vi "InstrumentSelection.vi"(8 "error in (no error)":errorcluster, 9 "Verify GPIB address":bool, 10 "Instrument type":T1(ring), 11 "Instrument name IN":string(combo)) -> (0 "error out":errorcluster, 1 "Instrument name OUT":string, 2 "LCR":refnum<class "LCRControl.lvclass">, 3 "Supply":refnum<class "SupplyControl.lvclass">, 4 "Switching":refnum<class "Switching.lvclass">, 5 "Multimeter":refnum<class "MultimeterControl.lvclass">)   [LabVIEW 2018, in "InstrControl.lvclass"]
uses:
  InstrControl.lvclass
  SupplyControl/SupplyControl.lvclass
  C:/Users/itk/Documents/itk-strip-sensor-qc/InstrControl/InstrControl.lvclass
  LCRControl/LCRControl.lvclass
  MultimeterControl/MultimeterControl.lvclass
  Switching/Switching.lvclass
  SupplyControl/Keithley 2410/KE2410.lvclass
  C:/Users/itk/Documents/itk-strip-sensor-qc/InstrControl/SupplyControl/SupplyControl.lvclass
  SupplyControl/Keithley 6517/KE6517.lvclass
  SupplyControl/Keithley 487/KE487.lvclass
  SupplyControl/Keithley 2657/KE2657A.lvclass
  SupplyControl/Keithley 236 & 237/KE236.lvclass
  LCRControl/WK6440B/WK6440B.lvclass
  C:/Users/itk/Documents/itk-strip-sensor-qc/InstrControl/LCRControl/LCRControl.lvclass
  LCRControl/WK6425/WK6425.lvclass
  MultimeterControl/Keithley 2000/KE2000.lvclass
  C:/Users/itk/Documents/itk-strip-sensor-qc/InstrControl/MultimeterControl/MultimeterControl.lvclass
  Switching/Pickering/Pickering.lvclass
  C:/Users/itk/Documents/itk-strip-sensor-qc/InstrControl/Switching/Switching.lvclass
  InstrumentSetup.vi
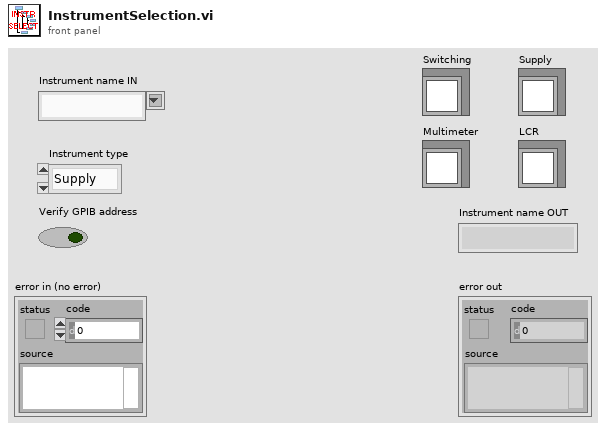
[diagram p1: front panel]
types:
  T1 = enum16{"Supply", "LCR", "Multimeter", "Switching"}
  T2 = cluster{"KE 2410":cluster{"Instrument name":string, "GPIB address":string, "Instrument type":u16}, "KE 6517":cluster{"Instrument name":string, "GPIB address":string, "Instrument type":u16}, "KE 487":cluster{"Instrument name":string, "GPIB address":string, "Instrument type":u16}, "KE 487_2":cluster{"Instrument name":string, "GPIB address":string, "Instrument type":u16}, "KE 236":cluster{"Instrument name":string, "GPIB address":string, "Instrument type":u16}, "WK 6440B":cluster{"Instrument name":string, "GPIB address":string, "Instrument type":u16}, "WK 6425":cluster{"Instrument name":string, "GPIB address":string, "Instrument type":u16}, "Pickering Matrix":cluster{"Instrument name":string, "GPIB address":string, "Instrument type":u16}, "KE 2000":cluster{"Instrument name":string, "GPIB address":string, "Instrument type":u16}, "KE 2657A":cluster{"Instrument name":string, "GPIB address":string, "Instrument type":u16}, "Prague Pickering Matrix":cluster{"Instrument name":string, "GPIB address":string, "Instrument type":u16}}
  T3 = cluster{"Current Limit":sgl, "KE2410":refnum<class "KE2410.lvclass">}
  T4 = cluster{"Current Limit":u16, "KE6517":refnum<class "KE6517.lvclass">}
  T5 = cluster{"Compliance":u16, "Range:":u16, "KE487":refnum<class "KE487.lvclass">}
  T6 = cluster{"Current Limit":sgl, "Compliance":u16, "Range:":u16, "KE2657A":refnum<class "KE2657A.lvclass">}
  T7 = cluster{"current \ncompliance level":dbl, "compliance/\nmeasurement range (auto:0)":u16, "KE236":refnum<class "KE236.lvclass">}
  T8 = cluster{"RC Configuration":u16, "AC amplitude [V]":dbl, "AC frequency [Hz]":i32, "WK6440B":refnum<class "WK6440B.lvclass">}
  T9 = cluster{"RC Configuration":u16, "AC amplitude [V]":dbl, "AC frequency [Hz]":i32, "WK6425":refnum<class "WK6425.lvclass">}
  T10 = cluster{"Range":u16, "Range Value":dbl, "Function":u16, "KE2000":refnum<class "KE2000.lvclass">}
  T11 = cluster{"Matrix address":string, "Mux1 address":string, "Mux2 address":string, "Matrix used?":bool, "Pickering":refnum<class "Pickering.lvclass">, "Matrix X Channels":cluster{"Bias Supply / SMU LO":i32, "Bias Supply / SMU HI":i32, "CV Box LO":i32, "CV Box HI":i32, "CV Box LO IN":i32, "CV Box HI IN":i32, "Volt meter LO":i32, "Volt meter HI":i32, "Mux1 C1":i32, "Mux1 C2":i32, "Mux2 C1":i32, "Mux2 C2":i32}}
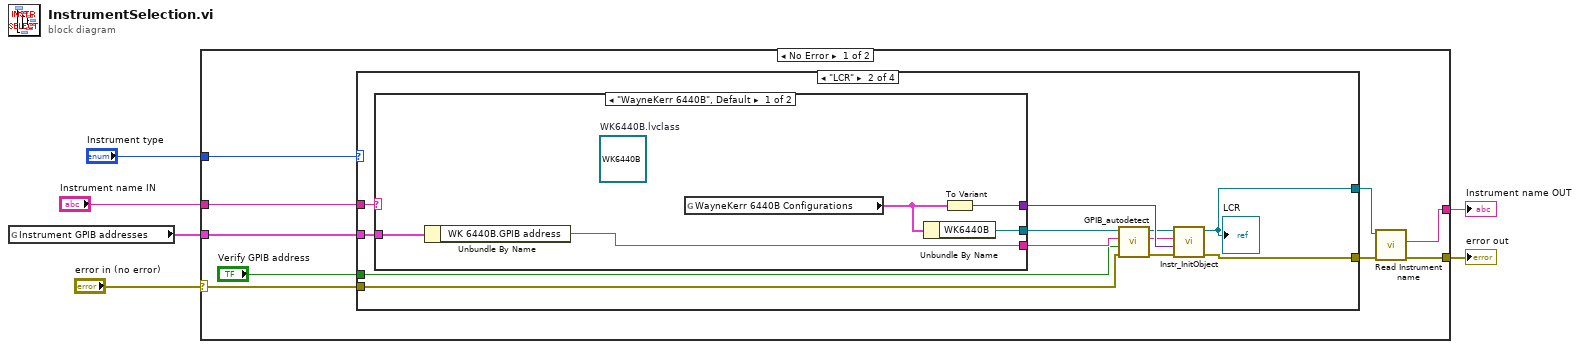
[diagram p0: block diagram]
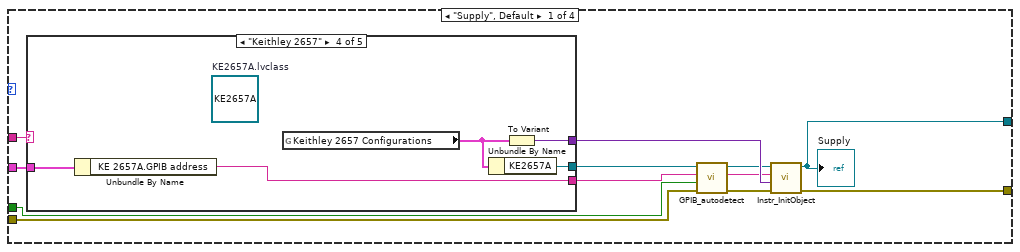
[diagram p2: hidden frame]
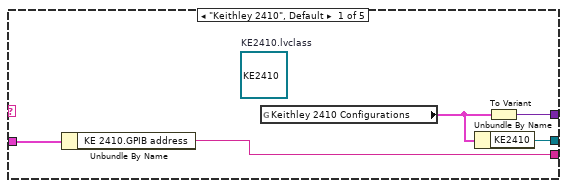
[diagram p3: hidden frame]
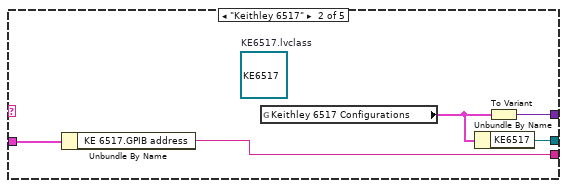
[diagram p4: hidden frame]
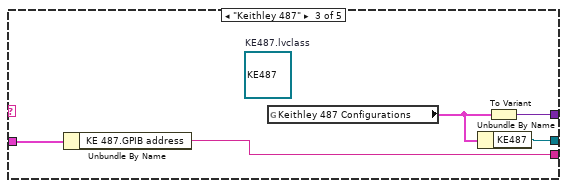
[diagram p5: hidden frame]
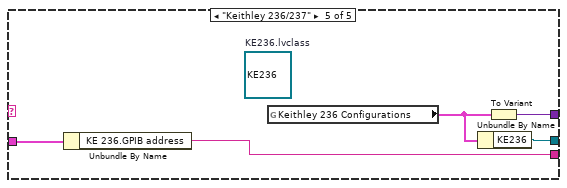
[diagram p6: hidden frame]
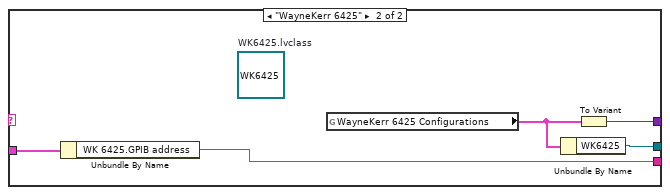
[diagram p7: hidden frame]
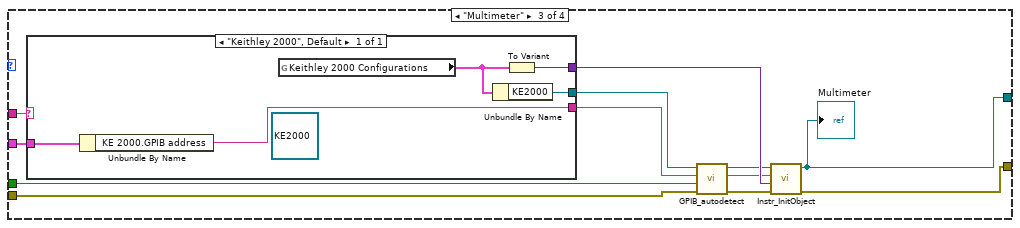
[diagram p8: hidden frame]
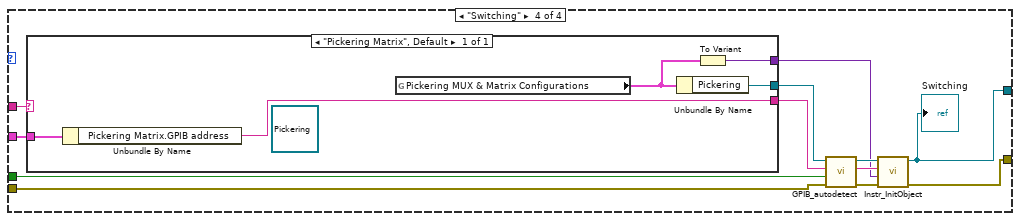
[diagram p9: hidden frame]
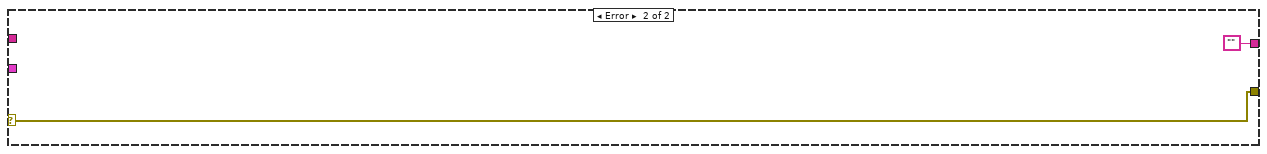
[diagram p10: hidden frame]
diagram:
  n1 = global read "InstrumentSetup.vi" "Instrument GPIB addresses"() -> (w1:T2)
  n2 = case shown="No Error" "error in (no error)" {
    selector: "error in (no error)" -> [w13 w110]
    tunnel: [w14 w110] -> w5
    tunnel: [w15 ""] -> w4
    tunnel: "Instrument type" -> [w10 _]
    tunnel: "Instrument name IN" -> [w9 _]
    tunnel: w1 -> [w8 _]
    frame No Error {
      n3 = case shown="\"LCR\"" w10 {
        tunnel: w9 -> [w27 w64 w86 w94]
        tunnel: [w26 w62 w84 w102] -> w12
        tunnel: w13 -> [w18 w59 w76 w96]
        tunnel: [w25 w63 w85 w103] -> w11
        tunnel: w8 -> [w24 w61 w83 w100]
        tunnel: "Verify GPIB address" -> [w17 w53 w81 w95]
        frame "Supply", Default {
          n4 = case shown="\"Keithley 2657\"" w27 {
            tunnel: [w29 w33 w38 w43 w48] -> w20
            tunnel: w24 -> [w32 w37 w42 w47 w52]
            tunnel: [w31 w36 w41 w46 w51] -> w22
            tunnel: [w30 w35 w40 w45 w50] -> w23
            frame "Keithley 2410", Default {
              (unwired) refnum<class "KE2410.lvclass"> refnum  # KE2410.lvclass
              n5 = Unbundle By Name(w32) -> ("KE 2410.GPIB address"=w31:string)
              n6 = global read "InstrumentSetup.vi" "Keithley 2410 Configurations"() -> (w28:T3)
              n7 = Unbundle By Name(w28) -> ("KE2410"=w29:refnum<class "KE2410.lvclass">)
              n8 = To Variant(anything=w28) -> (Variant=w30:variant)
            }
            frame "Keithley 6517" {
              (unwired) refnum<class "KE6517.lvclass"> refnum  # KE6517.lvclass
              n9 = Unbundle By Name(w37) -> ("KE 6517.GPIB address"=w36:string)
              n10 = global read "InstrumentSetup.vi" "Keithley 6517 Configurations"() -> (w34:T4)
              n11 = Unbundle By Name(w34) -> ("KE6517"=w33:refnum<class "KE6517.lvclass">)
              n12 = To Variant(anything=w34) -> (Variant=w35:variant)
            }
            frame "Keithley 487" {
              (unwired) refnum<class "KE487.lvclass"> refnum  # KE487.lvclass
              n13 = Unbundle By Name(w42) -> ("KE 487.GPIB address"=w41:string)
              n14 = global read "InstrumentSetup.vi" "Keithley 487 Configurations"() -> (w39:T5)
              n15 = Unbundle By Name(w39) -> ("KE487"=w38:refnum<class "KE487.lvclass">)
              n16 = To Variant(anything=w39) -> (Variant=w40:variant)
            }
            frame "Keithley 2657" {
              (unwired) refnum<class "KE2657A.lvclass"> refnum  # KE2657A.lvclass
              n17 = Unbundle By Name(w47) -> ("KE 2657A.GPIB address"=w46:string)
              n18 = global read "InstrumentSetup.vi" "Keithley 2657 Configurations"() -> (w44:T6)
              n19 = Unbundle By Name(w44) -> ("KE2657A"=w43:refnum<class "KE2657A.lvclass">)
              n20 = To Variant(anything=w44) -> (Variant=w45:variant)
            }
            frame "Keithley 236/237" {
              (unwired) refnum<class "KE236.lvclass"> refnum  # KE236.lvclass
              n21 = Unbundle By Name(w52) -> ("KE 236.GPIB address"=w51:string)
              n22 = global read "InstrumentSetup.vi" "Keithley 236 Configurations"() -> (w49:T7)
              n23 = Unbundle By Name(w49) -> ("KE236"=w48:refnum<class "KE236.lvclass">)
              n24 = To Variant(anything=w49) -> (Variant=w50:variant)
            }
          }
          n25 = call-dynamic "GPIB_autodetect.vi"("error in (no error)"=w18, "Verify GPIB address"=w17, "Instrument GPIB address in"=w22, "InstrControl in"=w20) -> ("error out"=w16:errorcluster, "Instrument GPIB address"=w21:string, "InstrControl out"=w19:refnum<class "SupplyControl.lvclass">)  [unwired: 5 in]
          n26 = call-dynamic "Instr_InitObject.vi"("error in (no error)"=w16, "Instrument Configuration"=w23, "GPIB address"=w21, "SupplyControl in"=w19) -> ("error out"=w25:errorcluster, "SupplyControl out"=w26:refnum<class "SupplyControl.lvclass">)  [unwired: 6 in]
          "Supply" <- w26
        }
        frame "LCR" {
          n27 = case shown="\"WayneKerr 6440B\", Default" w64 {
            tunnel: [w65 w70] -> w55
            tunnel: w61 -> [w69 w74]
            tunnel: [w68 w73] -> w57
            tunnel: [w67 w72] -> w60
            frame "WayneKerr 6440B", Default {
              (unwired) refnum<class "WK6440B.lvclass"> refnum  # WK6440B.lvclass
              n28 = Unbundle By Name(w69) -> ("WK 6440B.GPIB address"=w68:string)
              n29 = global read "InstrumentSetup.vi" "WayneKerr 6440B Configurations"() -> (w66:T8)
              n30 = Unbundle By Name(w66) -> ("WK6440B"=w65:refnum<class "WK6440B.lvclass">)
              n31 = To Variant(anything=w66) -> (Variant=w67:variant)
            }
            frame "WayneKerr 6425" {
              (unwired) refnum<class "WK6425.lvclass"> refnum  # WK6425.lvclass
              n32 = Unbundle By Name(w74) -> ("WK 6425.GPIB address"=w73:string)
              n33 = global read "InstrumentSetup.vi" "WayneKerr 6425 Configurations"() -> (w71:T9)
              n34 = Unbundle By Name(w71) -> ("WK6425"=w70:refnum<class "WK6425.lvclass">)
              n35 = To Variant(anything=w71) -> (Variant=w72:variant)
            }
          }
          n36 = call-dynamic "GPIB_autodetect.vi"("error in (no error)"=w59, "Verify GPIB address"=w53, "Instrument GPIB address in"=w57, "InstrControl in"=w55) -> ("error out"=w58:errorcluster, "Instrument GPIB address"=w56:string, "InstrControl out"=w54:refnum<class "LCRControl.lvclass">)  [unwired: 5 in]
          n37 = call-dynamic "Instr_InitObject.vi"("error in (no error)"=w58, "Instrument Configuration"=w60, "GPIB Address"=w56, "LCRControl in"=w54) -> ("error out"=w63:errorcluster, "LCRControl out"=w62:refnum<class "LCRControl.lvclass">)  [unwired: 6 in]
          "LCR" <- w62
        }
        frame "Multimeter" {
          n38 = case shown="\"Keithley 2000\", Default" w86 {
            tunnel: [w87] -> w77
            tunnel: w83 -> [w91]
            tunnel: [w90] -> w80
            tunnel: [w89] -> w82
            frame "Keithley 2000", Default {
              (unwired) refnum<class "KE2000.lvclass"> refnum ("KE2000.lvclass")
              n39 = Unbundle By Name(w91) -> ("KE 2000.GPIB address"=w90:string)
              n40 = global read "InstrumentSetup.vi" "Keithley 2000 Configurations"() -> (w88:T10)
              n41 = Unbundle By Name(w88) -> ("KE2000"=w87:refnum<class "KE2000.lvclass">)
              n42 = To Variant(anything=w88) -> (Variant=w89:variant)
            }
          }
          n43 = call-dynamic "GPIB_autodetect.vi"("error in (no error)"=w76, "Verify GPIB address"=w81, "Instrument GPIB address in"=w80, "InstrControl in"=w77) -> ("error out"=w75:errorcluster, "Instrument GPIB address"=w79:string, "InstrControl out"=w78:refnum<class "KE2000.lvclass">)  [unwired: 5 in]
          n44 = call-dynamic "Instr_InitObject.vi"("error in (no error)"=w75, "Instrument Configuration"=w82, "GPIB Address"=w79, "KE2000 in"=w78) -> ("error out"=w85:errorcluster, "KE2000 out"=w84:refnum<class "KE2000.lvclass">)  [unwired: 6 in]
          "Multimeter" <- w84
        }
        frame "Switching" {
          n45 = case shown="\"Pickering Matrix\", Default" w94 {
            tunnel: w100 -> [w108]
            tunnel: [w107] -> w99
            tunnel: [w105] -> w93
            tunnel: [w104] -> w92
            frame "Pickering Matrix", Default {
              (unwired) refnum<class "Pickering.lvclass"> refnum ("Pickering")
              n46 = Unbundle By Name(w108) -> ("Pickering Matrix.GPIB address"=w107:string)
              n47 = global read "InstrumentSetup.vi" "Pickering MUX & Matrix Configurations"() -> (w106:T11)
              n48 = Unbundle By Name(w106) -> ("Pickering"=w104:refnum<class "Pickering.lvclass">)
              n49 = To Variant(anything=w106) -> (Variant=w105:variant)
            }
          }
          n50 = call-dynamic "GPIB_autodetect.vi"("error in (no error)"=w96, "Verify GPIB address"=w95, "Instrument GPIB address in"=w99, "InstrControl in"=w92) -> ("error out"=w98:errorcluster, "Instrument GPIB address"=w97:string, "InstrControl out"=w101:refnum<class "Pickering.lvclass">)  [unwired: 5 in]
          n51 = call-dynamic "Instr_InitObject.vi"("error in (no error)"=w98, "Instrument Configuration"=w93, "GPIB Address"=w97, "Pickering in"=w101) -> ("error out"=w103:errorcluster, "Pickering out"=w102:refnum<class "Pickering.lvclass">)  [unwired: 6 in]
          "Switching" <- w102
        }
      }
      n52 = call-dynamic "Read Instrument name.vi"("error in (no error)"=w11, "InstControl in"=w12) -> ("error out"=w14:errorcluster, "Instrument name"=w15:string)  [unwired: 7 in, 1 out]
    }
    frame Error {
    }
  }
  "error out" <- w5
  "Instrument name OUT" <- w4
